vi "MotorOpen.vi"(8 "error in (no error)":errorcluster, 11 "RobotConfigIn":T1={"Motors"={"RightDrivePrimary"={"CAN Address"=0, "Invert"=FALSE, "InvertSensor"=FALSE, "Unit Conversion Factor"=0.0, "Brake Mode"=enum."Override to Brake", "Reverse Limt Switch Mode"=enum."Disabled", "Forward Limt Swith Mode"=enum."Disabled", "PWM Channel"=enum."Invalid", "Motor Controller Type"=enum."Talon SRX", "Peak Current (A)"=0, "Continuous Current (A)"=0, "Peak Duration (ms)"=0, "Current Limit Enable"=FALSE}, "RightDriveSecondary"={"CAN Address"=0, "Invert"=FALSE, "InvertSensor"=FALSE, "Unit Conversion Factor"=0.0, "Brake Mode"=enum."Override to Brake", "Reverse Limt Switch Mode"=enum."Disabled", "Forward Limt Swith Mode"=enum."Disabled", "PWM Channel"=enum."Invalid", "Motor Controller Type"=enum."Talon SRX", "Peak Current (A)"=0, "Continuous Current (A)"=0, "Peak Duration (ms)"=0, "Current Limit Enable"=FALSE}, "LeftDrivePrimary"={"CAN Address"=0, "Invert"=FALSE, "InvertSensor"=FALSE, "Unit Conversion Factor"=0.0, "Brake Mode"=enum."Override to Brake", "Reverse Limt Switch Mode"=enum."Disabled", "Forward Limt Swith Mode"=enum."Disabled", "PWM Channel"=enum."Invalid", "Motor Controller Type"=enum."Talon SRX", "Peak Current (A)"=0, "Continuous Current (A)"=0, "Peak Duration (ms)"=0, "Current Limit Enable"=FALSE}, "LeftDriveSecondary"={"CAN Address"=0, "Invert"=FALSE, "InvertSensor"=FALSE, "Unit Conversion Factor"=0.0, "Brake Mode"=enum."Override to Brake", "Reverse Limt Switch Mode"=enum."Disabled", "Forward Limt Swith Mode"=enum."Disabled", "PWM Channel"=enum."Invalid", "Motor Controller Type"=enum."Talon SRX", "Peak Current (A)"=0, "Continuous Current (A)"=0, "Peak Duration (ms)"=0, "Current Limit Enable"=FALSE}, "RightShooter"={"CAN Address"=0, "Invert"=FALSE, "InvertSensor"=FALSE, "Unit Conversion Factor"=0.0, "Brake Mode"=enum."Override to Brake", "Reverse Limt Switch Mode"=enum."Disabled", "Forward Limt Swith Mode"=enum."Disabled", "PWM Channel"=enum."Invalid", "Motor Controller Type"=enum."Talon SRX", "Peak Current (A)"=0, "Continuous Current (A)"=0, "Peak Duration (ms)"=0, "Current Limit Enable"=FALSE}, "LeftShooter"={"CAN Address"=0, "Invert"=FALSE, "InvertSensor"=FALSE, "Unit Conversion Factor"=0.0, "Brake Mode"=enum."Override to Brake", "Reverse Limt Switch Mode"=enum."Disabled", "Forward Limt Swith Mode"=enum."Disabled", "PWM Channel"=enum."Invalid", "Motor Controller Type"=enum."Talon SRX", "Peak Current (A)"=0, "Continuous Current (A)"=0, "Peak Duration (ms)"=0, "Current Limit Enable"=FALSE}, "ShooterRotate"={"CAN Address"=0, "Invert"=FALSE, "InvertSensor"=FALSE, "Unit Conversion Factor"=0.0, "Brake Mode"=enum."Override to Brake", "Reverse Limt Switch Mode"=enum."Disabled", "Forward Limt Swith Mode"=enum."Disabled", "PWM Channel"=enum."Invalid", "Motor Controller Type"=enum."Talon SRX", "Peak Current (A)"=0, "Continuous Current (A)"=0, "Peak Duration (ms)"=0, "Current Limit Enable"=FALSE}, "ShooterHood"={"CAN Address"=0, "Invert"=FALSE, "InvertSensor"=FALSE, "Unit Conversion Factor"=0.0, "Brake Mode"=enum."Override to Brake", "Reverse Limt Switch Mode"=enum."Disabled", "Forward Limt Swith Mode"=enum."Disabled", "PWM Channel"=enum."Invalid", "Motor Controller Type"=enum."Talon SRX", "Peak Current (A)"=0, "Continuous Current (A)"=0, "Peak Duration (ms)"=0, "Current Limit Enable"=FALSE}, "HopperWheel"={"CAN Address"=0, "Invert"=FALSE, "InvertSensor"=FALSE, "Unit Conversion Factor"=0.0, "Brake Mode"=enum."Override to Brake", "Reverse Limt Switch Mode"=enum."Disabled", "Forward Limt Swith Mode"=enum."Disabled", "PWM Channel"=enum."Invalid", "Motor Controller Type"=enum."Talon SRX", "Peak Current (A)"=0, "Continuous Current (A)"=0, "Peak Duration (ms)"=0, "Current Limit Enable"=FALSE}, "Elevator"={"CAN Address"=0, "Invert"=FALSE, "InvertSensor"=FALSE, "Unit Conversion Factor"=0.0, "Brake Mode"=enum."Override to Brake", "Reverse Limt Switch Mode"=enum."Disabled", "Forward Limt Swith Mode"=enum."Disabled", "PWM Channel"=enum."Invalid", "Motor Controller Type"=enum."Talon SRX", "Peak Current (A)"=0, "Continuous Current (A)"=0, "Peak Duration (ms)"=0, "Current Limit Enable"=FALSE}, "ClimberRaise"={"CAN Address"=0, "Invert"=FALSE, "InvertSensor"=FALSE, "Unit Conversion Factor"=0.0, "Brake Mode"=enum."Override to Brake", "Reverse Limt Switch Mode"=enum."Disabled", "Forward Limt Swith Mode"=enum."Disabled", "PWM Channel"=enum."Invalid", "Motor Controller Type"=enum."Talon SRX", "Peak Current (A)"=0, "Continuous Current (A)"=0, "Peak Duration (ms)"=0, "Current Limit Enable"=FALSE}, "ClimberPullUp"={"CAN Address"=0, "Invert"=FALSE, "InvertSensor"=FALSE, "Unit Conversion Factor"=0.0, "Brake Mode"=enum."Override to Brake", "Reverse Limt Switch Mode"=enum."Disabled", "Forward Limt Swith Mode"=enum."Disabled", "PWM Channel"=enum."Invalid", "Motor Controller Type"=enum."Talon SRX", "Peak Current (A)"=0, "Continuous Current (A)"=0, "Peak Duration (ms)"=0, "Current Limit Enable"=FALSE}, "Intake"={"CAN Address"=0, "Invert"=FALSE, "InvertSensor"=FALSE, "Unit Conversion Factor"=0.0, "Brake Mode"=enum."Override to Brake", "Reverse Limt Switch Mode"=enum."Disabled", "Forward Limt Swith Mode"=enum."Disabled", "PWM Channel"=enum."Invalid", "Motor Controller Type"=enum."Talon SRX", "Peak Current (A)"=0, "Continuous Current (A)"=0, "Peak Duration (ms)"=0, "Current Limit Enable"=FALSE}, "ControlPanel"={"CAN Address"=0, "Invert"=FALSE, "InvertSensor"=FALSE, "Unit Conversion Factor"=0.0, "Brake Mode"=enum."Override to Brake", "Reverse Limt Switch Mode"=enum."Disabled", "Forward Limt Swith Mode"=enum."Disabled", "PWM Channel"=enum."Invalid", "Motor Controller Type"=enum."Talon SRX", "Peak Current (A)"=0, "Continuous Current (A)"=0, "Peak Duration (ms)"=0, "Current Limit Enable"=FALSE}}, "PID"={"Shooter"={"P"=0.0, "I"=0.0, "D"=0.0, "F"=0.0, "IZone"=0.0}, "Turret"={"P"=0.0, "I"=0.0, "D"=0.0, "F"=0.0, "IZone"=0.0}, "Elevator"={"P"=0.0, "I"=0.0, "D"=0.0, "F"=0.0, "IZone"=0.0}, "ControlPanel"={"P"=0.0, "I"=0.0, "D"=0.0, "F"=0.0, "IZone"=0.0}}, "MotionMagic"={"Turret"={"CruiseVelocity"=0, "Acceleration"=0}, "Elevator"={"CruiseVelocity"=0, "Acceleration"=0}, "ControlPanel"={"CruiseVelocity"=0, "Acceleration"=0}}, "Sensors"={"IMU"={"Yaw Axis"=enum."Z", "SPI Bus"=enum."SPI MXP", "AHRS Algorithm"=enum."Complementary", "Calibration Time (s)"=3.0, "Calibrate On Open"=TRUE}, "ElevatorBottom"={"ID"=0, "RangingMode"=enum."Short", "sampleTime(ms)"=24.0}, "ElevatorTop"={"ID"=0, "RangingMode"=enum."Short", "sampleTime(ms)"=24.0}}, "Solenoids"={"Intake"={"SolenoidChannel"=enum."Solenoid 0", "Invert"=FALSE}}, "EnableCompressor"=FALSE, "RobotDimensions"={"Wheelbase(in)"=0.0, "Length(in)"=0.0}, "CameraMounting"={"LensHeight(in)"=0.0, "RotationRadius(in)"=0.0, "Pitch(deg)"=0.0}} {"Sensors"."ElevatorTop"."sampleTime(ms)" min=24.0 max=1000.0 step=1.0; "Sensors"."ElevatorBottom"."sampleTime(ms)" min=24.0 max=1000.0 step=1.0}) -> (0 "error out":errorcluster, 3 "RobotConfigOut":T1={"Motors"={"RightDrivePrimary"={"CAN Address"=0, "Invert"=FALSE, "InvertSensor"=FALSE, "Unit Conversion Factor"=0.0, "Brake Mode"=enum."Override to Brake", "Reverse Limt Switch Mode"=enum."Disabled", "Forward Limt Swith Mode"=enum."Disabled", "PWM Channel"=enum."Invalid", "Motor Controller Type"=enum."Talon SRX", "Peak Current (A)"=0, "Continuous Current (A)"=0, "Peak Duration (ms)"=0, "Current Limit Enable"=FALSE}, "RightDriveSecondary"={"CAN Address"=0, "Invert"=FALSE, "InvertSensor"=FALSE, "Unit Conversion Factor"=0.0, "Brake Mode"=enum."Override to Brake", "Reverse Limt Switch Mode"=enum."Disabled", "Forward Limt Swith Mode"=enum."Disabled", "PWM Channel"=enum."Invalid", "Motor Controller Type"=enum."Talon SRX", "Peak Current (A)"=0, "Continuous Current (A)"=0, "Peak Duration (ms)"=0, "Current Limit Enable"=FALSE}, "LeftDrivePrimary"={"CAN Address"=0, "Invert"=FALSE, "InvertSensor"=FALSE, "Unit Conversion Factor"=0.0, "Brake Mode"=enum."Override to Brake", "Reverse Limt Switch Mode"=enum."Disabled", "Forward Limt Swith Mode"=enum."Disabled", "PWM Channel"=enum."Invalid", "Motor Controller Type"=enum."Talon SRX", "Peak Current (A)"=0, "Continuous Current (A)"=0, "Peak Duration (ms)"=0, "Current Limit Enable"=FALSE}, "LeftDriveSecondary"={"CAN Address"=0, "Invert"=FALSE, "InvertSensor"=FALSE, "Unit Conversion Factor"=0.0, "Brake Mode"=enum."Override to Brake", "Reverse Limt Switch Mode"=enum."Disabled", "Forward Limt Swith Mode"=enum."Disabled", "PWM Channel"=enum."Invalid", "Motor Controller Type"=enum."Talon SRX", "Peak Current (A)"=0, "Continuous Current (A)"=0, "Peak Duration (ms)"=0, "Current Limit Enable"=FALSE}, "RightShooter"={"CAN Address"=0, "Invert"=FALSE, "InvertSensor"=FALSE, "Unit Conversion Factor"=0.0, "Brake Mode"=enum."Override to Brake", "Reverse Limt Switch Mode"=enum."Disabled", "Forward Limt Swith Mode"=enum."Disabled", "PWM Channel"=enum."Invalid", "Motor Controller Type"=enum."Talon SRX", "Peak Current (A)"=0, "Continuous Current (A)"=0, "Peak Duration (ms)"=0, "Current Limit Enable"=FALSE}, "LeftShooter"={"CAN Address"=0, "Invert"=FALSE, "InvertSensor"=FALSE, "Unit Conversion Factor"=0.0, "Brake Mode"=enum."Override to Brake", "Reverse Limt Switch Mode"=enum."Disabled", "Forward Limt Swith Mode"=enum."Disabled", "PWM Channel"=enum."Invalid", "Motor Controller Type"=enum."Talon SRX", "Peak Current (A)"=0, "Continuous Current (A)"=0, "Peak Duration (ms)"=0, "Current Limit Enable"=FALSE}, "ShooterRotate"={"CAN Address"=0, "Invert"=FALSE, "InvertSensor"=FALSE, "Unit Conversion Factor"=0.0, "Brake Mode"=enum."Override to Brake", "Reverse Limt Switch Mode"=enum."Disabled", "Forward Limt Swith Mode"=enum."Disabled", "PWM Channel"=enum."Invalid", "Motor Controller Type"=enum."Talon SRX", "Peak Current (A)"=0, "Continuous Current (A)"=0, "Peak Duration (ms)"=0, "Current Limit Enable"=FALSE}, "ShooterHood"={"CAN Address"=0, "Invert"=FALSE, "InvertSensor"=FALSE, "Unit Conversion Factor"=0.0, "Brake Mode"=enum."Override to Brake", "Reverse Limt Switch Mode"=enum."Disabled", "Forward Limt Swith Mode"=enum."Disabled", "PWM Channel"=enum."Invalid", "Motor Controller Type"=enum."Talon SRX", "Peak Current (A)"=0, "Continuous Current (A)"=0, "Peak Duration (ms)"=0, "Current Limit Enable"=FALSE}, "HopperWheel"={"CAN Address"=0, "Invert"=FALSE, "InvertSensor"=FALSE, "Unit Conversion Factor"=0.0, "Brake Mode"=enum."Override to Brake", "Reverse Limt Switch Mode"=enum."Disabled", "Forward Limt Swith Mode"=enum."Disabled", "PWM Channel"=enum."Invalid", "Motor Controller Type"=enum."Talon SRX", "Peak Current (A)"=0, "Continuous Current (A)"=0, "Peak Duration (ms)"=0, "Current Limit Enable"=FALSE}, "Elevator"={"CAN Address"=0, "Invert"=FALSE, "InvertSensor"=FALSE, "Unit Conversion Factor"=0.0, "Brake Mode"=enum."Override to Brake", "Reverse Limt Switch Mode"=enum."Disabled", "Forward Limt Swith Mode"=enum."Disabled", "PWM Channel"=enum."Invalid", "Motor Controller Type"=enum."Talon SRX", "Peak Current (A)"=0, "Continuous Current (A)"=0, "Peak Duration (ms)"=0, "Current Limit Enable"=FALSE}, "ClimberRaise"={"CAN Address"=0, "Invert"=FALSE, "InvertSensor"=FALSE, "Unit Conversion Factor"=0.0, "Brake Mode"=enum."Override to Brake", "Reverse Limt Switch Mode"=enum."Disabled", "Forward Limt Swith Mode"=enum."Disabled", "PWM Channel"=enum."Invalid", "Motor Controller Type"=enum."Talon SRX", "Peak Current (A)"=0, "Continuous Current (A)"=0, "Peak Duration (ms)"=0, "Current Limit Enable"=FALSE}, "ClimberPullUp"={"CAN Address"=0, "Invert"=FALSE, "InvertSensor"=FALSE, "Unit Conversion Factor"=0.0, "Brake Mode"=enum."Override to Brake", "Reverse Limt Switch Mode"=enum."Disabled", "Forward Limt Swith Mode"=enum."Disabled", "PWM Channel"=enum."Invalid", "Motor Controller Type"=enum."Talon SRX", "Peak Current (A)"=0, "Continuous Current (A)"=0, "Peak Duration (ms)"=0, "Current Limit Enable"=FALSE}, "Intake"={"CAN Address"=0, "Invert"=FALSE, "InvertSensor"=FALSE, "Unit Conversion Factor"=0.0, "Brake Mode"=enum."Override to Brake", "Reverse Limt Switch Mode"=enum."Disabled", "Forward Limt Swith Mode"=enum."Disabled", "PWM Channel"=enum."Invalid", "Motor Controller Type"=enum."Talon SRX", "Peak Current (A)"=0, "Continuous Current (A)"=0, "Peak Duration (ms)"=0, "Current Limit Enable"=FALSE}, "ControlPanel"={"CAN Address"=0, "Invert"=FALSE, "InvertSensor"=FALSE, "Unit Conversion Factor"=0.0, "Brake Mode"=enum."Override to Brake", "Reverse Limt Switch Mode"=enum."Disabled", "Forward Limt Swith Mode"=enum."Disabled", "PWM Channel"=enum."Invalid", "Motor Controller Type"=enum."Talon SRX", "Peak Current (A)"=0, "Continuous Current (A)"=0, "Peak Duration (ms)"=0, "Current Limit Enable"=FALSE}}, "PID"={"Shooter"={"P"=0.0, "I"=0.0, "D"=0.0, "F"=0.0, "IZone"=0.0}, "Turret"={"P"=0.0, "I"=0.0, "D"=0.0, "F"=0.0, "IZone"=0.0}, "Elevator"={"P"=0.0, "I"=0.0, "D"=0.0, "F"=0.0, "IZone"=0.0}, "ControlPanel"={"P"=0.0, "I"=0.0, "D"=0.0, "F"=0.0, "IZone"=0.0}}, "MotionMagic"={"Turret"={"CruiseVelocity"=0, "Acceleration"=0}, "Elevator"={"CruiseVelocity"=0, "Acceleration"=0}, "ControlPanel"={"CruiseVelocity"=0, "Acceleration"=0}}, "Sensors"={"IMU"={"Yaw Axis"=enum."Z", "SPI Bus"=enum."SPI MXP", "AHRS Algorithm"=enum."Complementary", "Calibration Time (s)"=3.0, "Calibrate On Open"=TRUE}, "ElevatorBottom"={"ID"=0, "RangingMode"=enum."Short", "sampleTime(ms)"=24.0}, "ElevatorTop"={"ID"=0, "RangingMode"=enum."Short", "sampleTime(ms)"=24.0}}, "Solenoids"={"Intake"={"SolenoidChannel"=enum."Solenoid 0", "Invert"=FALSE}}, "EnableCompressor"=FALSE, "RobotDimensions"={"Wheelbase(in)"=0.0, "Length(in)"=0.0}, "CameraMounting"={"LensHeight(in)"=0.0, "RotationRadius(in)"=0.0, "Pitch(deg)"=0.0}} {"Sensors"."ElevatorTop"."sampleTime(ms)" min=24.0 max=1000.0 step=1.0; "Sensors"."ElevatorBottom"."sampleTime(ms)" min=24.0 max=1000.0 step=1.0})   [LabVIEW 2019]
uses:
  TypeDefs/ConfigComponents/Config_Robot.ctl
  ArgosLib/Config/ConfigComponents/TypeDefs/Config_Motor.ctl
  <vilib>/Rock Robotics/WPI/ThirdParty/Phoenix-LabVIEW/Motor Controller/Controls/CTRE_Phoenix_MotorControl_NeutralMode.ctl
  <vilib>/Rock Robotics/WPI/ThirdParty/Phoenix-LabVIEW/Motor Controller/Controls/CTRE_Phoenix_MotorControl_LimitSwitchNormal.ctl
  <vilib>/Rock Robotics/SystemInterfaces/DIO/FPGA_DIOPWMChannel.ctl
  ArgosLib/Config/ConfigComponents/TypeDefs/Config_MotorCtrlType.ctl
  ArgosLib/Config/ConfigComponents/TypeDefs/Config_PIDParams.ctl
  ArgosLib/Config/ConfigComponents/TypeDefs/Config_MotionMagicParams.ctl
  ArgosLib/Config/ConfigComponents/TypeDefs/Config_IMU.ctl
  <vilib>/Rock Robotics/SystemInterfaces/spilib/spi_bus.ctl
  ArgosLib/Config/ConfigComponents/TypeDefs/Config_PwFToF.ctl
  <vilib>/Playing With Fusion Inc/Playing With Fusion Lib for FRC/PWF_ToF_LabVIEW/Public/TypeDefs/PwF_ToF_RangingMode.ctl
  ArgosLib/Config/ConfigComponents/TypeDefs/Config_SingleSolenoid.ctl
  <vilib>/Rock Robotics/WPI/Solenoid/WPI_SolenoidChannel.ctl
  TypeDefs/ConfigComponents/Config_RobotDimensions.ctl
  TypeDefs/ConfigComponents/Config_CameraMounting.ctl
  ArgosLib/Drive/MotorControl/RobotDriveOpen6MotorWithVenom.vi
  ArgosLib/Drive/MotorControl/RobotDriveOpen6MotorWithTalonSRX.vi
  ArgosLib/Drive/MotorControl/RobotDriveOpen6MotorWithTalonSR.vi
  ArgosLib/ArgosLib.lvlib
  <vilib>/Playing With Fusion Inc/Playing With Fusion Lib for FRC/PWF_ToF_LabVIEW/PwF_ToF.lvlib
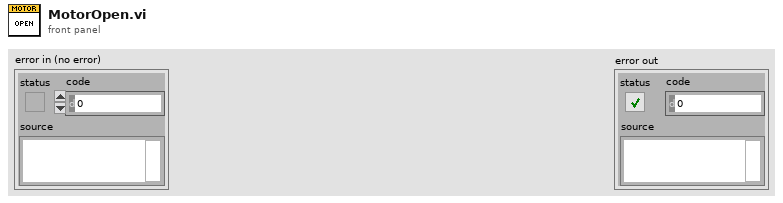
[diagram p1: front panel]
types:
  T1 = typedef "Config_Robot.ctl" = cluster{"Motors":cluster{"RightDrivePrimary":T2, "RightDriveSecondary":T2, "LeftDrivePrimary":T2, "LeftDriveSecondary":T2, "RightShooter":T2, "LeftShooter":T2, "ShooterRotate":T2, "ShooterHood":T2, "HopperWheel":T2, "Elevator":T2, "ClimberRaise":T2, "ClimberPullUp":T2, "Intake":T2, "ControlPanel":T2}, "PID":cluster{"Shooter":T7, "Turret":T7, "Elevator":T7, "ControlPanel":T7}, "MotionMagic":cluster{"Turret":T8, "Elevator":T8, "ControlPanel":T8}, "Sensors":cluster{"IMU":T9, "ElevatorBottom":T11, "ElevatorTop":T11}, "Solenoids":cluster{"Intake":T13}, "EnableCompressor":bool, "RobotDimensions":T15, "CameraMounting":T16}
  T2 = typedef "ArgosLib.lvlib/Config_Motor.ctl" = cluster{"CAN Address":u8, "Invert":bool, "InvertSensor":bool, "Unit Conversion Factor":dbl, "Brake Mode":T3, "Reverse Limt Switch Mode":T4, "Forward Limt Swith Mode":T4, "PWM Channel":T5, "Motor Controller Type":T6, "Peak Current (A)":i32, "Continuous Current (A)":i32, "Peak Duration (ms)":i32, "Current Limit Enable":bool}
  T3 = typedef "CTRE_Phoenix_MotorControl_NeutralMode.ctl" = enum8{"EEPROMSetting", "Override to Coast", "Override to Brake"}
  T4 = typedef "CTRE_Phoenix_MotorControl_LimitSwitchNormal.ctl" = enum16{"Normally Open", "Normally Closed", "Disabled"}
  T5 = typedef "FPGA_DIOPWMChannel.ctl" = enum8{"PWM 0", "PWM 1", "PWM 2", "PWM 3", "PWM 4", "PWM 5", "PWM 6", "PWM 7", "PWM 8", "PWM 9", "PWM MXP 0", "PWM MXP 1", "PWM MXP 2", "PWM MXP 3", "PWM MXP 4", "PWM MXP 5", "PWM MXP 6", "PWM MXP 7", "PWM MXP 8", "PWM MXP 9", "Invalid"}
  T6 = typedef "ArgosLib.lvlib/Config_MotorCtrlType.ctl" = enum16{"Disabled", "Talon SRX", "Talon SR", "Venom", "Spark MAX"}
  T7 = typedef "ArgosLib.lvlib/Config_PIDParams.ctl" = cluster{"P":dbl, "I":dbl, "D":dbl, "F":dbl, "IZone":dbl}
  T8 = typedef "ArgosLib.lvlib/Config_MotionMagicParams.ctl" = cluster{"CruiseVelocity":i32, "Acceleration":i32}
  T9 = typedef "ArgosLib.lvlib/Config_IMU.ctl" = cluster{"Yaw Axis":enum16{"X", "Y", "Z"}, "SPI Bus":T10, "AHRS Algorithm":enum16{"Complementary", "Madgwick"}, "Calibration Time (s)":dbl, "Calibrate On Open":bool}
  T10 = typedef "spi_bus.ctl" = enum16{"SPI On-Board, CS0", "SPI On-Board, CS1", "SPI On-Board, CS2", "SPI On-Board, CS3", "SPI MXP", "Invalid"}
  T11 = typedef "ArgosLib.lvlib/Config_PwFToF.ctl" = cluster{"ID":u8, "RangingMode":T12, "sampleTime(ms)":dbl}
  T12 = typedef "PlayingWithFusionLib.lvlib/PwF_ToF.lvlib/PwF_ToF_RangingMode.ctl" = enum16{"Short", "Medium", "Long"}
  T13 = typedef "ArgosLib.lvlib/Config_SingleSolenoid.ctl" = cluster{"SolenoidChannel":T14, "Invert":bool}
  T14 = typedef "WPI_SolenoidChannel.ctl" = enum8{"Solenoid 0", "Solenoid 1", "Solenoid 2", "Solenoid 3", "Solenoid 4", "Solenoid 5", "Solenoid 6", "Solenoid 7", "Invalid"}
  T15 = typedef "Config_RobotDimensions.ctl" = cluster{"Wheelbase(in)":dbl, "Length(in)":dbl}
  T16 = typedef "Config_CameraMounting.ctl" = cluster{"LensHeight(in)":dbl, "RotationRadius(in)":dbl, "Pitch(deg)":dbl}
  T17 = typedef "WPI_MotorControlDeviceRef.ctl" = cluster{"DeviceStatus":errorcluster, "Type":T18, "PWM":cluster{"PWM Channel":T5, "DeadBand":T19}, "CAN":cluster{"Device Number":u8, "SetOutput VI Ref":variant, "GetOutput VI Ref":variant, "Enable VI Ref":variant, "Disable VI Ref":variant, "Data":variant}, "Invert":bool, "DIO PWM":cluster{"PWM \"Enable\" Channel":T5, "DIOChannel":T20, "PWM Rate":dbl}}
  T18 = typedef "WPI_MotorControlType.ctl" = enum16{"PWM", "CAN", "DIO PWM"}
  T19 = typedef "WPI_PWMDeadband.ctl" = cluster{"Name":string, "maxPositivePwm":i32, "minPositivePwm":i32, "centerPwm":i32, "maxNegativePwm":i32, "minNegativePwm":i32, "angularRange":u16}
  T20 = typedef "FPGA_DIOChannel.ctl" = enum8{"DIO 0", "DIO 1", "DIO 2", "DIO 3", "DIO 4", "DIO 5", "DIO 6", "DIO 7", "DIO 8", "DIO 9", "DIO MXP 0", "DIO MXP 1", "DIO MXP 2", "DIO MXP 3", "DIO MXP 4", "DIO MXP 5", "DIO MXP 6", "DIO MXP 7", "DIO MXP 8", "DIO MXP 9", "DIO MXP 10", "DIO MXP 11", "DIO MXP 12", "DIO MXP 13", "DIO MXP 14", "DIO MXP 15", "SPI Port CS1", "SPI Port CS2", "SPI Port CS3", "SPI Port MISO", "SPI Port MOSI", "Invalid"}
  T21 = typedef "WPI_RobotDriveDevRef.ctl" = cluster{"DevStatus":errorcluster, "Motors[]":T17[], "Square Inputs":bool, "Max Output":dbl}
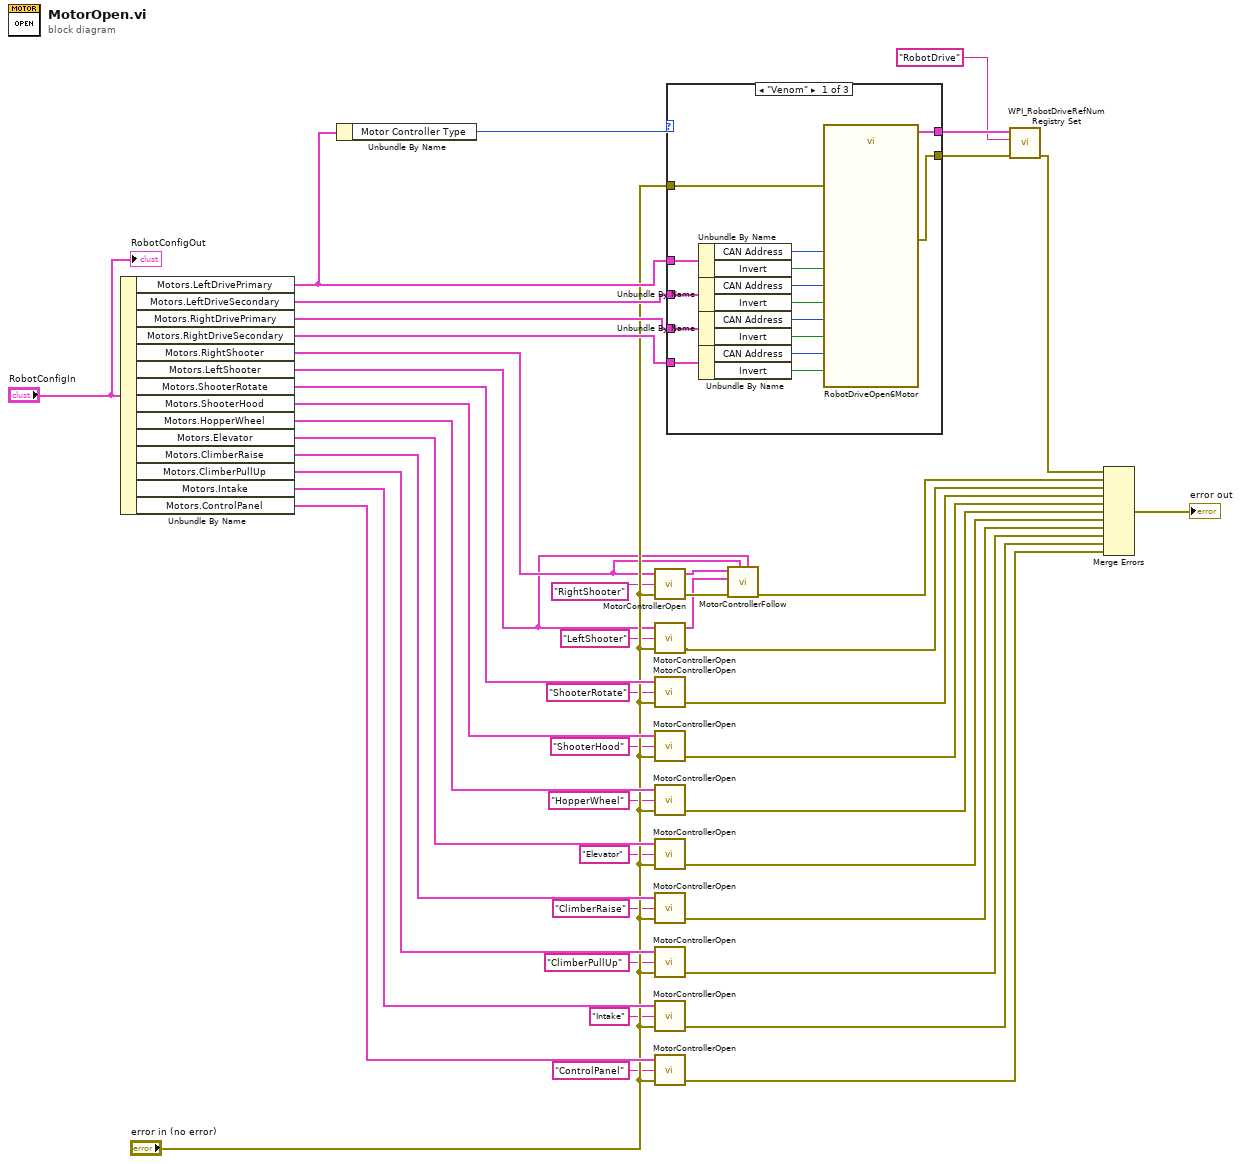
[diagram p0: block diagram]
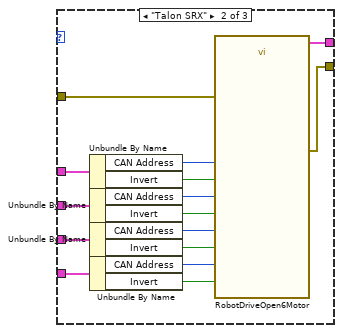
[diagram p2: hidden frame]
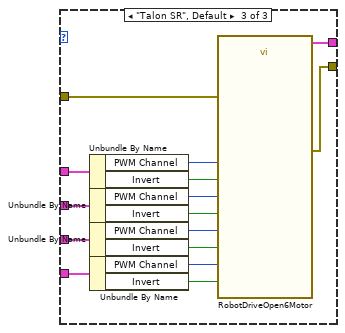
[diagram p3: hidden frame]
diagram:
  n1 = Unbundle By Name("RobotConfigIn") -> ("Motors.LeftDrivePrimary"=w41:T2, "Motors.LeftDriveSecondary"=w40:T2, "Motors.RightDrivePrimary"=w39:T2, "Motors.RightDriveSecondary"=w38:T2, "Motors.RightShooter"=w2:T2, "Motors.LeftShooter"=w1:T2, "Motors.ShooterRotate"=w37:T2, "Motors.ShooterHood"=w36:T2, "Motors.HopperWheel"=w35:T2, "Motors.Elevator"=w34:T2, "Motors.ClimberRaise"=w33:T2, "Motors.ClimberPullUp"=w32:T2, "Motors.Intake"=w31:T2, "Motors.ControlPanel"=w30:T2)
  n2 = Unbundle By Name(w41) -> ("Motor Controller Type"=w44:T6)
  n3 = call "MotorControllerOpen.vi"("error in"="error in (no error)", "RefnumName"="RightShooter", "MotorConfig"=w2) -> ("error out"=w5:errorcluster, "MotorControlDevRef"=w6:T17)  [unwired: 1 in]
  n4 = call "MotorControllerOpen.vi"("error in"="error in (no error)", "RefnumName"="LeftShooter", "MotorConfig"=w1) -> ("error out"=w7:errorcluster, "MotorControlDevRef"=w3:T17)  [unwired: 1 in]
  n5 = call "MotorControllerOpen.vi"("error in"="error in (no error)", "RefnumName"="ShooterRotate", "MotorConfig"=w37) -> ("error out"=w27:errorcluster)  [unwired: 1 in, 1 out]
  n6 = call "MotorControllerOpen.vi"("error in"="error in (no error)", "RefnumName"="ShooterHood", "MotorConfig"=w36) -> ("error out"=w26:errorcluster)  [unwired: 1 in, 1 out]
  n7 = call "MotorControllerOpen.vi"("error in"="error in (no error)", "RefnumName"="HopperWheel", "MotorConfig"=w35) -> ("error out"=w25:errorcluster)  [unwired: 1 in, 1 out]
  n8 = call "MotorControllerOpen.vi"("error in"="error in (no error)", "RefnumName"="Elevator", "MotorConfig"=w34) -> ("error out"=w24:errorcluster)  [unwired: 1 in, 1 out]
  n9 = call "MotorControllerOpen.vi"("error in"="error in (no error)", "RefnumName"="ClimberRaise", "MotorConfig"=w33) -> ("error out"=w23:errorcluster)  [unwired: 1 in, 1 out]
  n10 = call "MotorControllerOpen.vi"("error in"="error in (no error)", "RefnumName"="ClimberPullUp", "MotorConfig"=w32) -> ("error out"=w22:errorcluster)  [unwired: 1 in, 1 out]
  n11 = call "MotorControllerOpen.vi"("error in"="error in (no error)", "RefnumName"="Intake", "MotorConfig"=w31) -> ("error out"=w21:errorcluster)  [unwired: 1 in, 1 out]
  n12 = call "MotorControllerOpen.vi"("error in"="error in (no error)", "RefnumName"="ControlPanel", "MotorConfig"=w30) -> ("error out"=w20:errorcluster)  [unwired: 1 in, 1 out]
  n13 = case shown="\"Venom\"" w44 {
    tunnel: [w60 w75 w90] -> w43
    tunnel: [w59 w74 w89] -> w42
    tunnel: w41 -> [w58 w73 w88]
    tunnel: w40 -> [w49 w64 w79]
    tunnel: w39 -> [w48 w63 w78]
    tunnel: w38 -> [w47 w62 w77]
    tunnel: "error in (no error)" -> [w46 w61 w76]
    frame "Venom" {
      n14 = Unbundle By Name(w58) -> ("CAN Address"=w57:u8, "Invert"=w56:bool)
      n15 = Unbundle By Name(w49) -> ("CAN Address"=w55:u8, "Invert"=w54:bool)
      n16 = Unbundle By Name(w48) -> ("CAN Address"=w53:u8, "Invert"=w52:bool)
      n17 = Unbundle By Name(w47) -> ("CAN Address"=w51:u8, "Invert"=w50:bool)
      n18 = call-poly "RobotDriveOpen6Motor.vi"("Left Motor 1"=w57, "Left Motor 2"=w55, "Right Motor 1"=w53, "Right Motor 2"=w51, "error in (no error)"=w46, "Left Motor 1 Inverted"=w56, "Right Motor 1 Inverted"=w52, "Left Motor 2 Inverted"=w54, "Right Motor 2 Inverted"=w50) -> ("RobotDriveDevRef"=w60:T21, "error out"=w59:errorcluster)  [unwired: 17 in]
    }
    frame "Talon SRX" {
      n19 = Unbundle By Name(w73) -> ("CAN Address"=w72:u8, "Invert"=w71:bool)
      n20 = Unbundle By Name(w64) -> ("CAN Address"=w70:u8, "Invert"=w69:bool)
      n21 = Unbundle By Name(w63) -> ("CAN Address"=w68:u8, "Invert"=w67:bool)
      n22 = Unbundle By Name(w62) -> ("CAN Address"=w66:u8, "Invert"=w65:bool)
      n23 = call-poly "RobotDriveOpen6Motor.vi"("Left Motor 1"=w72, "Left Motor 2"=w70, "Right Motor 1"=w68, "Right Motor 2"=w66, "error in (no error)"=w61, "Left Motor 1 Inverted"=w71, "Right Motor 1 Inverted"=w67, "Left Motor 2 Inverted"=w69, "Right Motor 2 Inverted"=w65) -> ("RobotDriveDevRef"=w75:T21, "error out"=w74:errorcluster)  [unwired: 17 in]
    }
    frame "Talon SR", Default {
      n24 = Unbundle By Name(w88) -> ("PWM Channel"=w87:T5, "Invert"=w86:bool)
      n25 = Unbundle By Name(w79) -> ("PWM Channel"=w85:T5, "Invert"=w84:bool)
      n26 = Unbundle By Name(w78) -> ("PWM Channel"=w83:T5, "Invert"=w82:bool)
      n27 = Unbundle By Name(w77) -> ("PWM Channel"=w81:T5, "Invert"=w80:bool)
      n28 = call-poly "RobotDriveOpen6Motor.vi"("Left Motor 1"=w87, "Left Motor 2"=w85, "Right Motor 1"=w83, "Right Motor 2"=w81, "error in (no error)"=w76, "Left Motor 1 Inverted"=w86, "Right Motor 1 Inverted"=w82, "Left Motor 2 Inverted"=w84, "Right Motor 2 Inverted"=w80) -> ("RobotDriveDevRef"=w90:T21, "error out"=w89:errorcluster)  [unwired: 17 in]
    }
  }
  n29 = call "MotorControllerFollow.vi"("LeaderConfig"=w1, "FollowerConfig"=w2, "error in (no error)"=w5, "LeaderDevRef"=w3, "FollowerDevRef"=w6) -> ("error out"=w4:errorcluster)  [unwired: 5 in, 1 out]
  n30 = call <vilib>:"WPI_RobotDriveRefNum Registry Set.vi"("error in (no error)"=w42, "refnum name"="RobotDrive", "RobotDriveDevRef"=w43) -> ("error out"=w28:errorcluster)  [unwired: 7 in, 1 out]
  n31 = Merge Errors(w28, w4, w7, w27, w26, w25, w24, w23, w22, w21, w20) -> (→"error out":errorcluster)
  "RobotConfigOut" <- "RobotConfigIn"
